vi "CsTool-QueryStatusAll.vi"(1 "Handle Cluster":T1) -> (0 "Status":i32)   [LabVIEW 2022 SP3]
doc: "This VI returns the current acquisition status of the CompuScope system identified by Handle Cluster, which is obtained by calling CsTool-GetSystem.vi.\n\nIf the call is successful, a positive or zero status code is returned. The possible status return values are:\n 0 - indicates that the system has finished acquiring data.\n 1 - indicates that the system is acquiring, but has not yet been triggered.\n 2 - indicates that the system is acquiring, and has been triggered.\n 3 - indicates that the system is transferring data.\n\nA negative number is an error code. A descriptive error string may be obtained by using CsTool-ErrorHandler.vi."
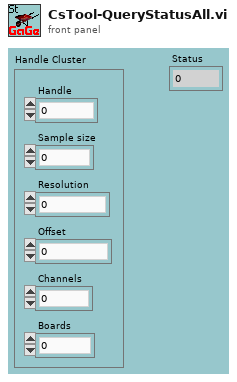
[diagram p1: front panel]
types:
  T1 = cluster{"Handle":u32, "Sample size":u32, "Resolution":i32, "Offset":i32, "Channels":u32, "Boards":u32}
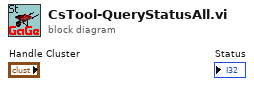
[diagram p0: block diagram]
diagram:
